vi "AVQ8347 Device Buzzer.vi"(8 "Error In":errorcluster, 10 "Buzzer Control (OFF)":bool, 11 "VISA Session":refnum<visa-resource-name>) -> (0 "Error Out":errorcluster, 2 "Send Code":string, 3 "Copy VISA Session":refnum<visa-resource-name>)   [LabVIEW 2018]
doc: "Control of buzzer sound"
panel:
  # "Device Buzzer"
  # "ON\nOFF"
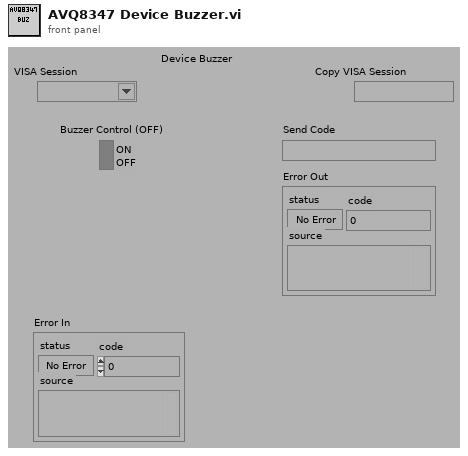
[diagram p1: front panel]
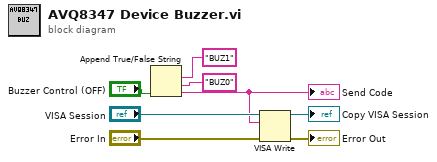
[diagram p0: block diagram]
diagram:
  n1 = Append True/False String(1:"Buzzer Control (OFF)", 2:"BUZ0", 3:"BUZ1") -> (0:w1:string)  [unwired: 1 in]
  "Send Code" <- w1
  n2 = VISA Write(VISA resource name="VISA Session", write buffer=w1, error in (no error)="Error In") -> (VISA resource name out=→"Copy VISA Session":refnum<visa-resource-name>, error out=→"Error Out":errorcluster)  [unwired: 1 out]
